vi "Update.vi"(8 "error in (no error)":errorcluster, 10 "Message in":refnum<class "UpdateMessage.lvclass">, 11 "ConfocalStage in":refnum<class "ConfocalStage.lvclass">) -> (0 "error out":errorcluster, 3 "ConfocalStage out":refnum<class "ConfocalStage.lvclass">)   [LabVIEW 2012, in "ConfocalStage.lvclass"]
doc: "The update method processes the command 'update'. \n\nThe command 'update' is used for receiving new values to be set to the private data of the class. This could be seen as a public set method for setting new parameters to the private class data."
uses:
  ConfocalStage.lvclass
  <vilib>/Distrio/Murmex/UpdateMessage/UpdateMessage.lvclass
  ConfocalStage.lvclass/ConfocalStage.ctl
  <vilib>/Distrio/Murmex/Murmex/Murmex.lvclass
panel:
  # "This method is called when the UPDATE\ntrigger is sent. \n\nOverride this method when your component needs to\nrespond to this trigger. \n\nCall parent for proper implementation"
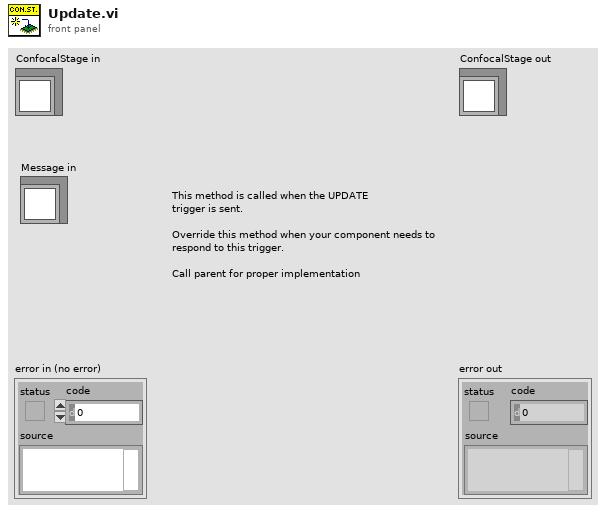
[diagram p1: front panel]
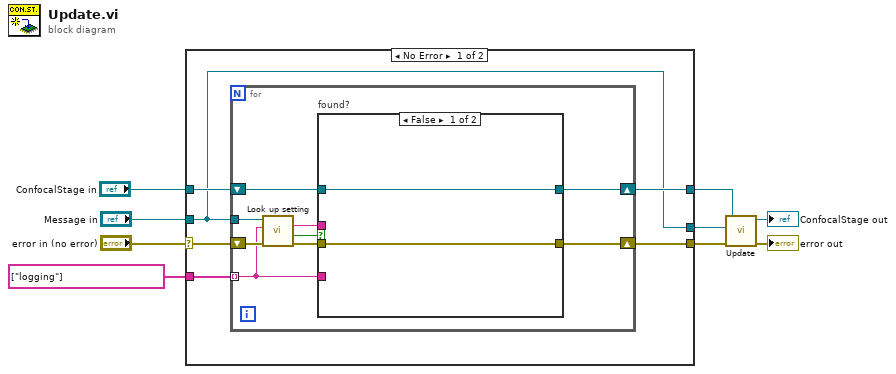
[diagram p0: block diagram]
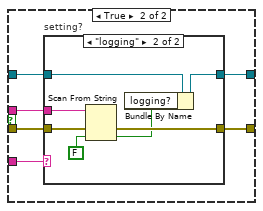
[diagram p2: hidden frame]
diagram:
  n1 = case shown="No Error" "error in (no error)" {
    selector: "error in (no error)" -> [w14 w44]
    tunnel: [w11 w44] -> w6
    tunnel: [w10 w43] -> w5
    tunnel: "Message in" -> [w10 w43]
    tunnel: [w12 w42] -> w3
    tunnel: "ConfocalStage in" -> [w13 w42]
    tunnel: string[] ["logging"] ("key chains") -> [w15 _]
    frame No Error {
      n2 = for {
        tunnel: w15 -> [w19] mode=indexing
        tunnel: w10 -> [w23]
        shift-right: [w18] -> w11
        shift-left: w14 -> [w24]
        shift-right: [w16] -> w12
        shift-left: w13 -> [w17]
        n3 = call <vilib>:"Look up setting.vi"("error in (no error)"=w24, "tag name"=w19, "UpdateMessage in"=w23) -> ("error out"=w21:errorcluster, "found?"=w22:bool, "value"=w20:string)  [unwired: 5 in, 1 out]
        n4 = case "found?" shown="False" w22 {
          tunnel: w21 -> [w25 w31]
          tunnel: w20 -> [_ w30]
          tunnel: w19 -> [_ w32]
          tunnel: [w25 w29] -> w18
          tunnel: w17 -> [w26 w28]
          tunnel: [w26 w27] -> w16
          frame False {
          }
          frame True {
            n5 = case "setting?" shown="\"logging\"" w32 {
              tunnel: w31 -> [w33 w40]
              tunnel: w30 -> [_ w39]
              tunnel: [w33 w38] -> w29
              tunnel: w28 -> [w34 w37]
              tunnel: [w34 w35] -> w27
              frame "False", Default {
              }
              frame "logging" {
                n6 = Scan From String(input string=w39, error in=w40, default 1=FALSE ("settings.logging?")) -> (error out=w38:errorcluster, output 1=w36:bool)  [unwired: 2 in, 2 out]
                n7 = Bundle By Name(cluster=w37, "logging?"=w36) -> (w35:refnum<class "ConfocalStage.lvclass">)
              }
            }
          }
        }
      }
    }
    frame Error {
    }
  }
  n8 = call-parent "Update.vi"("error in (no error)"=w6, "Message in"=w5, "Murmex in"=w3) -> ("error out"=→"error out":errorcluster, "Murmex out"=→"ConfocalStage out":refnum<class "ConfocalStage.lvclass">)  [unwired: 7 in]
